vi "Calibrate.vi"(8 "error in (no error)":errorcluster, 9 "Objects":T1[](array[typedef]) {"Aspect Ratio" format="%.2f"}) -> (0 "error out":errorcluster, 6 "Calibrated?":bool)   [LabVIEW 2015]
uses:
  TypeDefs Host/Object Info.ctl
  TypeDefs Host/Open Audio FGV Enum.ctl
  Kinect Support/Controls/Led Control.ctl
  TypeDefs Host/Counter FGV Enum.ctl
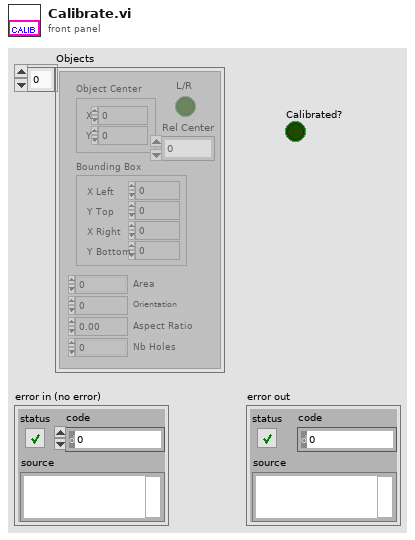
[diagram p1: front panel]
types:
  T1 = typedef "Object Info.ctl" = cluster{"Object Center":cluster{"X":u16, "Y":u16}, "Bounding Box":cluster{"X Left":u16, "Y Top":u16, "X Right":u16, "Y Bottom":u16}, "Area":u16, "Orientation":u16, "Aspect Ratio":sgl, "Nb Holes":u16, "L/R":bool, "Rel Center":u16}
  T2 = typedef "Open Audio FGV Enum.ctl" = enum16{"Get", "Set"}
  T3 = typedef "Led Control.ctl" = enum32{"LED_OFF", "LED_GREEN", "LED_RED", "LED_YELLOW", "LED_BLINK_GREEN", "LED_BLINK_GREEN2", "LED_BLINK_RED_YELLOW"}
  T4 = typedef "Counter FGV Enum.ctl" = enum16{"Get Count", "Set Count"}
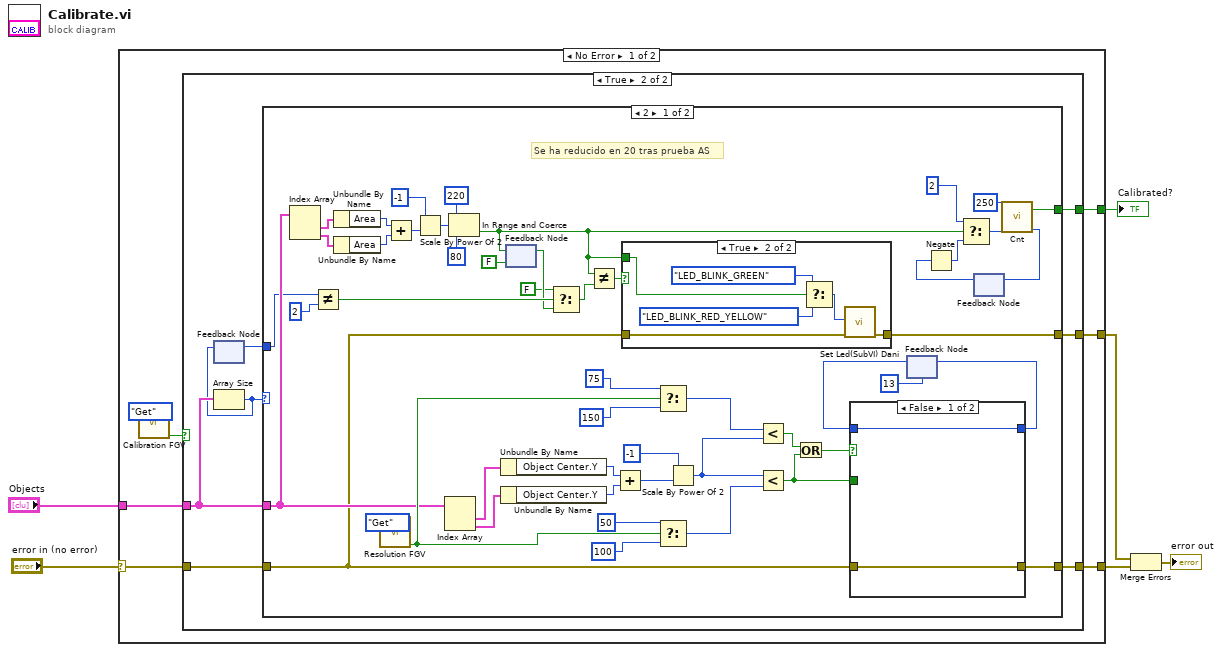
[diagram p0: block diagram]
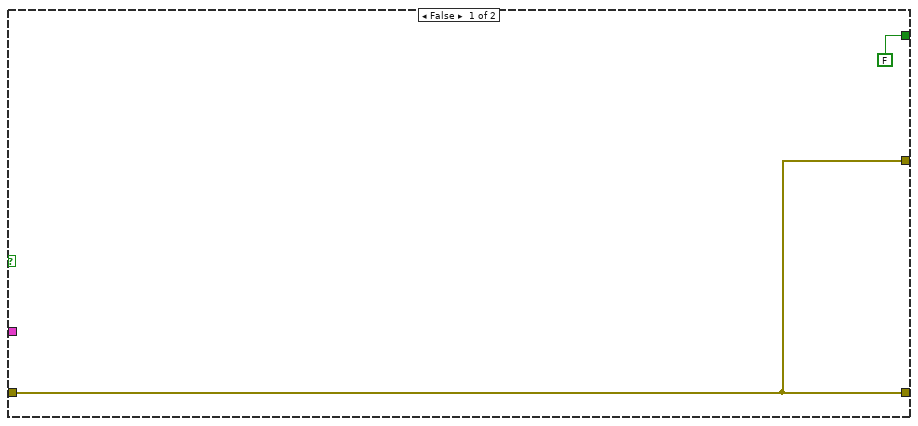
[diagram p2: hidden frame]
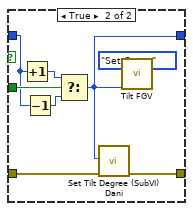
[diagram p4: hidden frame]
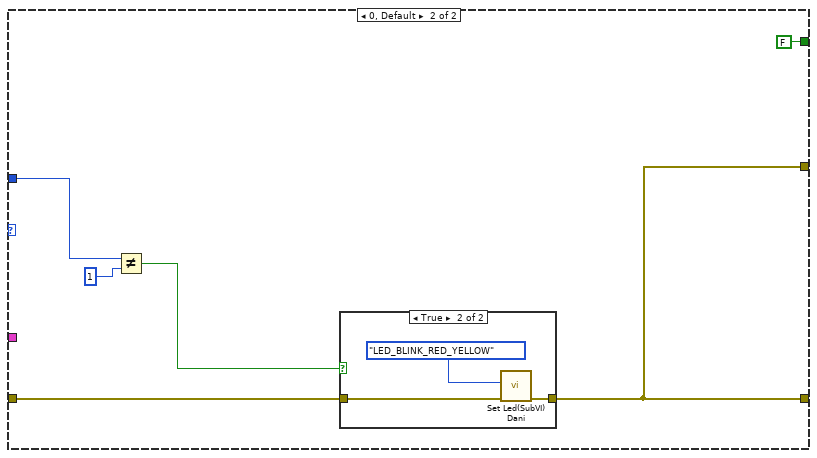
[diagram p5: hidden frame]
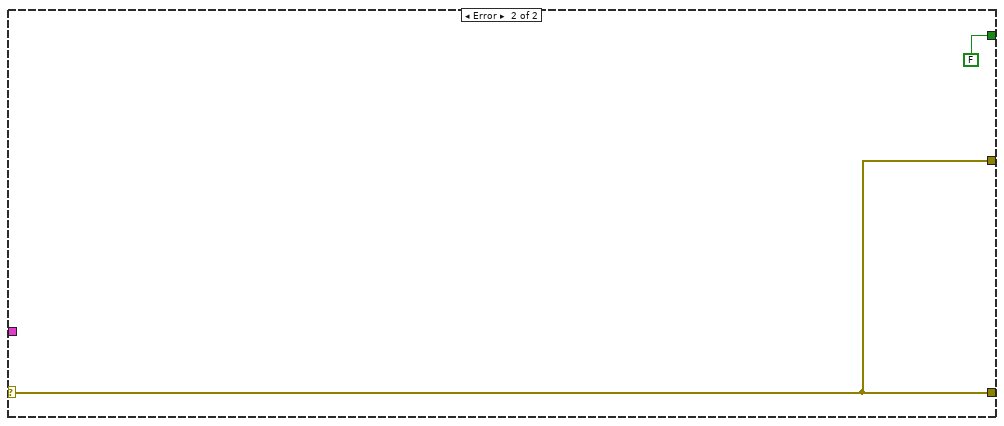
[diagram p7: hidden frame]
diagram:
  n1 = case shown="No Error" "error in (no error)" {
    selector: "error in (no error)" -> [w12 w100]
    tunnel: "Objects" -> [w11 _]
    tunnel: [w13 w100] -> w5
    tunnel: [w8 FALSE ("end")] -> w3
    tunnel: [w7 w100] -> w1
    frame No Error {
      n2 = call "Calibration FGV.vi"("Command"=Open_Audio_FGV_Enum."Get") -> ("Calib?"=w10:bool)  [unwired: 10 in]
      n3 = case shown="True" w10 {
        tunnel: [w14 w22] -> w13
        tunnel: w12 -> [w14 w21]
        tunnel: w11 -> [_ w20]
        tunnel: [FALSE ("end") w19] -> w8
        tunnel: [w14 w18] -> w7
        frame False {
        }
        frame True {
          n4 = feedback #1() -> (w16:i32)  [unwired: 1 in]
          n5 = Array Size(array=w20) -> (size(s)=w17:i32)
          n6 = feedback-in #1(w17) -> ()
          n7 = case shown="2" w17 {
            tunnel: w21 -> [w33 w94]
            tunnel: [w66 w93] -> w22
            tunnel: w20 -> [w36 _]
            tunnel: [w35 FALSE ("end")] -> w19
            tunnel: [w32 w93] -> w18
            tunnel: w16 -> [w27 w92]
            frame 2 {
              # "Se ha reducido en 20 tras prueba AS"
              n8 = Index Array(array=w36) -> (element #1=w40:T1, element #2=w41:T1)  [unwired: 2 in]
              n9 = Not Equal?(x=w27, y=2) -> (x != y?=w25:bool)
              n10 = Unbundle By Name(w40) -> ("Area"=w42:u16)
              n11 = Unbundle By Name(w41) -> ("Area"=w43:u16)
              n12 = call "Resolution FGV.vi"("Command"=Open_Audio_FGV_Enum."Get") -> ("L/T?"=w52:bool)  [unwired: 10 in]
              n13 = Add(x=w42, y=w43) -> (x+y=w44:u16)
              n14 = Scale By Power Of 2(n=i16 -1, x=w44) -> (x*2^n=w46:u16)
              n15 = Index Array(array=w36) -> (element #1=w72:T1, element #2=w71:T1)  [unwired: 2 in]
              n16 = In Range and Coerce(upper limit=u16 220, x=w46, lower limit=u16 80) -> (In Range?=w31:bool)  [unwired: 1 out]
              n17 = Unbundle By Name(w72) -> ("Object Center.Y"=w70:u16)
              n18 = Unbundle By Name(w71) -> ("Object Center.Y"=w69:u16)
              n19 = feedback-in #2(w31) -> ()
              n20 = feedback #2(FALSE) -> (w24:bool)
              n21 = Select(t=FALSE, s=w25, f=w24) -> (s? t:f=w28:bool)
              n22 = Not Equal?(x=w31, y=w28) -> (x != y?=w34:bool)
              n23 = Add(x=w70, y=w69) -> (x+y=w68:u16)
              n24 = case shown="True" w34 {
                tunnel: w33 -> [w73 w79]
                tunnel: [w73 w78] -> w32
                tunnel: w31 -> [_ w76]
                frame False {
                }
                frame True {
                  n25 = Select(t=Led_Control."LED_BLINK_GREEN" ("Led Option"), s=w76, f=Led_Control."LED_BLINK_RED_YELLOW" ("Led Option")) -> (s? t:f=w77:T3)
                  n26 = call "Set Led(SubVI) Dani.vi"("error in (no error)"=w79, "Led Option"=w77) -> ("error out"=w78:errorcluster)  [unwired: 9 in]
                }
              }
              n27 = Select(t=u16 75 ("altura max"), s=w52, f=u16 150 ("altura max")) -> (s? t:f=w57:u16)
              n28 = Select(t=u16 50 ("altura min"), s=w52, f=u16 100 ("altura min")) -> (s? t:f=w55:u16)
              n29 = Scale By Power Of 2(n=i16 -1, x=w68) -> (x*2^n=w65:u16)
              n30 = Less?(x=w57, y=w65) -> (x < y?=w64:bool)
              n31 = Less?(x=w65, y=w55) -> (x < y?=w61:bool)
              n32 = Or(x=w64, y=w61) -> (x .or. y?=w63:bool)
              n33 = feedback #3(13 ("degree")) -> (w60:i32)
              n34 = case shown="False" w63 {
                tunnel: w33 -> [w81 w89]
                tunnel: [w81 w88] -> w66
                tunnel: w61 -> [_ w87]
                tunnel: w60 -> [w80 w85]
                tunnel: [w80 w83] -> w59
                frame False {
                }
                frame True {
                  n35 = Increment(x=w85) -> (x+1=w86:i32)
                  n36 = Decrement(x=w85) -> (x-1=w84:i32)
                  n37 = Select(t=w86, s=w87, f=w84) -> (s? t:f=w83:i32)
                  n38 = call "Set Tilt Degree (SubVI) Dani.vi"("degree"=w83, "error in (no error)"=w89) -> ("error out"=w88:errorcluster)  [unwired: 8 in]
                  n39 = call "Tilt FGV.vi"("Exit FGV Command"=Counter_FGV_Enum."Set Count", "Tilt In"=w83) -> ()  [unwired: 9 in, 1 out]
                }
              }
              n40 = feedback-in #3(w59) -> ()
              n41 = feedback #4() -> (w37:i32)  [unwired: 1 in]
              n42 = Negate(x=w37) -> (-x=w49:i32)
              n43 = Select(t=2 ("f"), s=w31, f=w49) -> (s? t:f=w38:i32)
              n44 = call "Cnt.vi"("n-1"=250, "inc"=w38) -> ("i"=w30:i32, "end"=w35:bool)  [unwired: 8 in]
              n45 = feedback-in #4(w30) -> ()
            }
            frame 0, Default {
              n46 = Not Equal?(x=w92, y=1) -> (x != y?=w90:bool)
              n47 = case shown="True" w90 {
                tunnel: w94 -> [w96 w99]
                tunnel: [w96 w98] -> w93
                frame False {
                }
                frame True {
                  n48 = call "Set Led(SubVI) Dani.vi"("error in (no error)"=w99, "Led Option"=Led_Control."LED_BLINK_RED_YELLOW") -> ("error out"=w98:errorcluster)  [unwired: 9 in]
                }
              }
            }
          }
        }
      }
    }
    frame Error {
    }
  }
  "Calibrated?" <- w3
  n49 = Merge Errors(w1, w5) -> (→"error out":errorcluster)
